vi "数据类型转换.vi"(1 "待处理数据":u8[](array[numeric])) -> (0 "输出簇":T1)   [LabVIEW 2014]
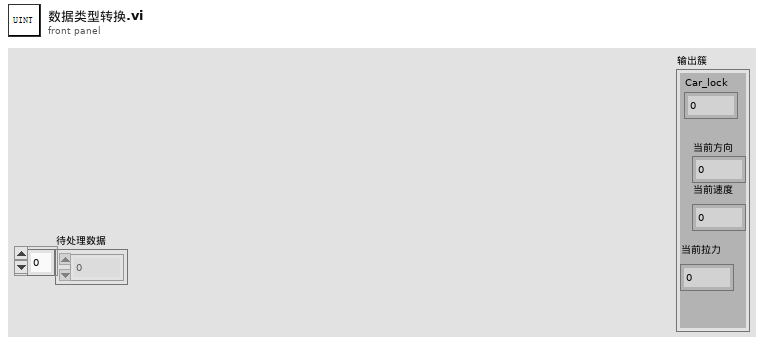
[diagram p1: front panel]
types:
  T1 = cluster{"Car_lock":u8, "当前方向":u8, "当前速度\n":u16, "当前拉力":u16}
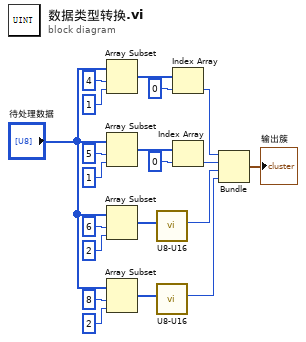
[diagram p0: block diagram]
diagram:
  n1 = Array Subset(array="待处理数据", index=4 ("长度（剩余）"), length=1 ("长度（剩余）")) -> (w11:u8[])
  n2 = Array Subset(array="待处理数据", index=5 ("长度（剩余）"), length=1 ("长度（剩余）")) -> (w8:u8[])
  n3 = Array Subset(array="待处理数据", index=6 ("长度（剩余）"), length=2 ("长度（剩余）")) -> (w5:u8[])
  n4 = Array Subset(array="待处理数据", index=8 ("长度（剩余）"), length=2 ("长度（剩余）")) -> (w1:u8[])
  n5 = call "U8-U16.vi"("数组"=w5) -> ("16位整型"=w15:u16)  [unwired: 8 in, 1 out]
  n6 = call "U8-U16.vi"("数组"=w1) -> ("16位整型"=w14:u16)  [unwired: 8 in, 1 out]
  n7 = Index Array(array=w11, index=0 ("索引")) -> (element=w18:u8)
  n8 = Index Array(array=w8, index=0 ("索引")) -> (element=w16:u8)
  n9 = Bundle(w18, w16, "16位整型"=w15, "16位整型"=w14) -> (→"输出簇":cluster{u8, u8, "16位整型":u16, "16位整型":u16})  [unwired: 1 in]
